vi "DB_Read.vi"(11 "Input Params":T1={"Address IP"="192.168.1.12", "Rack"=0, "Slot "=2, "DB Number"=1, "Start"=0, "Amount"=0}) -> (1 "?":string, 2 "Data":u8[](array[numeric]), 3 "Status":string="No Error")   [LabVIEW 2023]
uses:
  snap7-full-1.4.0/LabVIEW/lib/Snap7.lvlib
panel:
  out "Size Get":i32
  out "Running":bool
  in  "?":bool
  # "DB Get"
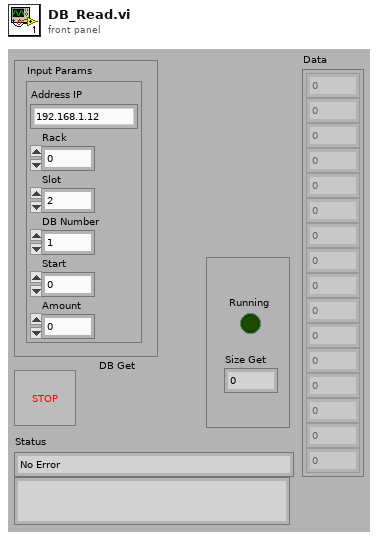
[diagram p1: front panel]
types:
  T1 = cluster{"Address IP":string, "Rack":i32, "Slot ":i32, "DB Number":i32, "Start":i32, "Amount":i32}
  T2 = enum16{"big-endian, network order", "native, host order", "little-endian"}
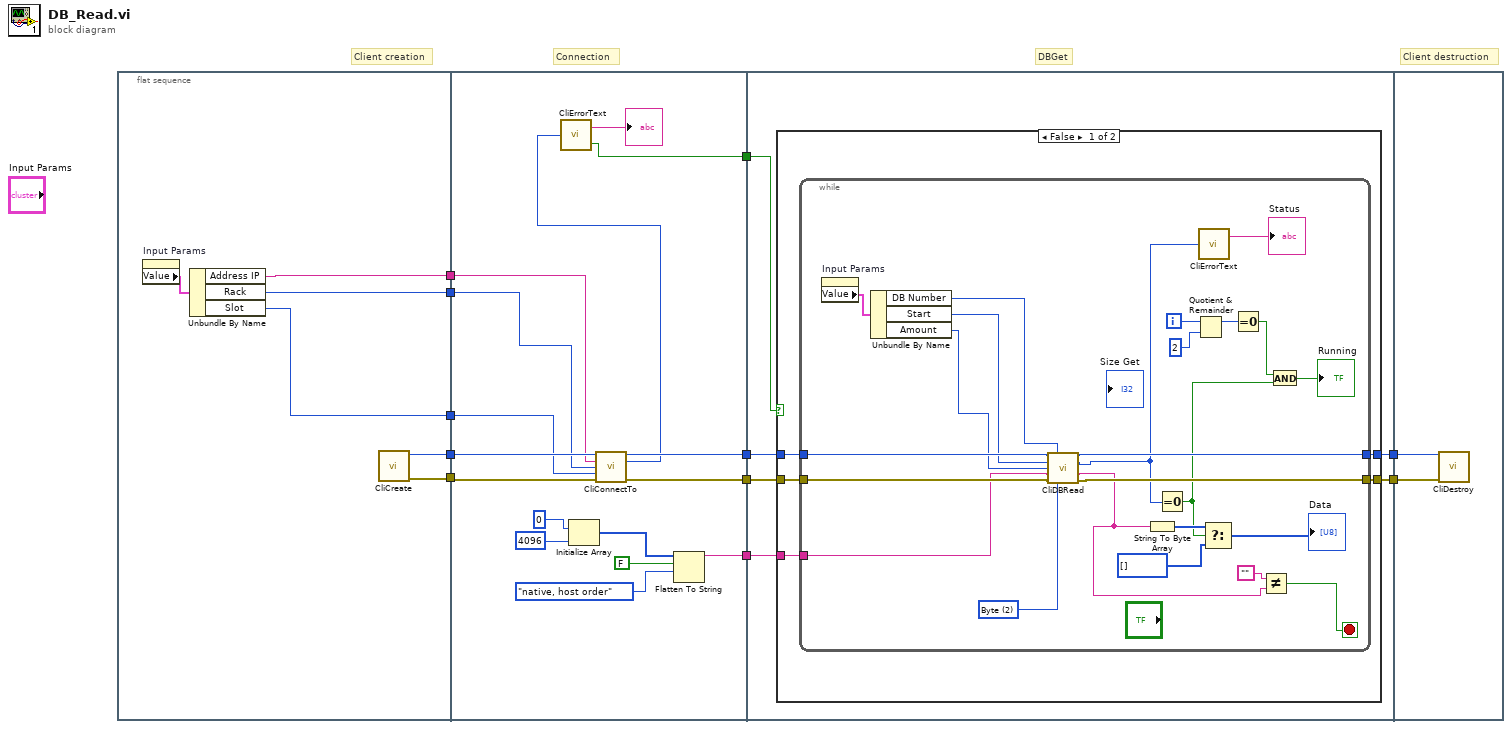
[diagram p0: block diagram]
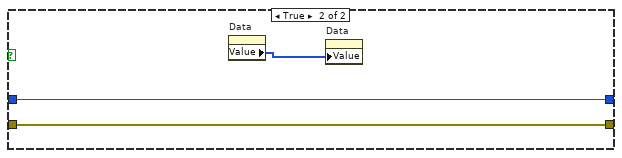
[diagram p2: hidden frame]
diagram:
  # "Client destruction"
  # "DBGet"
  # "Connection"
  # "Client creation"
  n1 = flat-sequence {
    tunnel: [w17] -> w8
    tunnel: [w16] -> w7
    tunnel: [w14] -> w4
    tunnel: [w13] -> w3
    tunnel: [w12] -> w2
    tunnel: [w28] -> w11
    tunnel: [w24] -> w10
    tunnel: [w27] -> w9
    tunnel: w8 -> [w26]
    tunnel: w7 -> [w25]
    tunnel: w4 -> [w21]
    tunnel: w3 -> [w20]
    tunnel: w2 -> [w19]
    tunnel: [w18] -> w1
    tunnel: w11 -> [w39]
    tunnel: w10 -> [w38]
    tunnel: w9 -> [w37]
    tunnel: [w36] -> w6
    tunnel: [w35] -> w5
    tunnel: w1 -> [w34]
    tunnel: w6 -> [w73]
    tunnel: w5 -> [w72]
    frame #0 {
      n2 = property on="Input Params" class="Clust (strict)"() -> ("Value"=w15:T1)  [unwired: 2 in, 2 out]
      n3 = Unbundle By Name(w15) -> ("Address IP"=w14:string, "Rack"=w13:i32, "Slot"=w12:i32)
      n4 = call "CliCreate.vi"() -> ("ref out"=w17:u64, "error out"=w16:errorcluster)  [unwired: 14 in]
    }
    frame #1 {
      n5 = Initialize Array(u8 0, 4096) -> (w31:u8[])
      n6 = call "CliConnectTo.vi"("ref in"=w26, "Address"=w21, "Rack"=w20, "Slot"=w19, "error in (no error)"=w25) -> ("ref out"=w24:u64, "Result"=w23:i32, "error out"=w28:errorcluster)  [unwired: 8 in]
      n7 = call "CliErrorText.vi"("ErrNo"=w23) -> ("Error"=w18:bool, "ErrMessage"=→"?":string)
      n8 = Flatten To String(anything=w31, prepend array or string size? (T)=FALSE, byte order (0:big-endian, network order)=T2."native, host order") -> (data string=w27:string)  [unwired: 1 in, 2 out]
    }
    frame #2 {
      n9 = case shown="False" w34 {
        tunnel: w39 -> [w44 w70]
        tunnel: w38 -> [w43 w71]
        tunnel: w37 -> [w42 _]
        tunnel: [w41 w71] -> w36
        tunnel: [w40 w70] -> w35
        frame False {
          n10 = while {
            tunnel: w44 -> [w60]
            tunnel: w43 -> [w58]
            tunnel: w42 -> [w59]
            tunnel: [w57] -> w41
            tunnel: [w56] -> w40
            i -> [w66]
            stop <- w48 stop-if-true
            w54 = 2 items=["Bit"=1, "Byte"=2, "Word"=4, "DWord"=6, "Real"=8, "Counter"=28, "Timer"=29] ("Word Length")
            n11 = property on="Input Params" class="Clust (strict)"() -> ("Value"=w53:T1)  [unwired: 2 in, 2 out]
            n12 = Unbundle By Name(w53) -> ("DB Number"=w52:i32, "Start"=w51:i32, "Amount"=w50:i32)
            n13 = call "CliDBRead.vi"("ref in"=w58, "DB Number"=w52, "Start"=w51, "Amount"=w50, "data in"=w59, "error in (no error)"=w60, "Word Length"=w54) -> ("ref out"=w57:u64, "Result"=w55:i32, "data out"=w46:string, "error out"=w56:errorcluster)  [unwired: 5 in]
            n14 = String To Byte Array(string=w46) -> (unsigned byte array=w68:u8[])
            n15 = Equal To 0?(x=w55) -> (x = 0?=w49:bool)
            n16 = Quotient & Remainder(x=w66, y=2) -> (x-y*floor(x/y)=w64:i32)  [unwired: 1 out]
            n17 = call "CliErrorText.vi"("ErrNo"=w55) -> ("ErrMessage"=→"Status":string)  [unwired: 1 out]
            n18 = Select(t=w68, s=w49, f=u8[] []) -> (s? t:f=→"Data":u8[])
            n19 = Equal To 0?(x=w64) -> (x = 0?=w63:bool)
            n20 = Not Equal?(x="", y=w46) -> (x != y?=w48:bool)
            n21 = And(x=w63, y=w49) -> (x .and. y?=→"Running":bool)
          }
        }
        frame True {
          n22 = property on="Data" class="Arr (strict)"() -> ("Value"=w69:u8[])  [unwired: 2 in, 2 out]
          n23 = property on="Data" class="Arr (strict)"("Value"=w69) -> ()  [unwired: 2 in, 2 out]
        }
      }
    }
    frame #3 {
      n24 = call "CliDestroy.vi"("ref in"=w73, "error in (no error)"=w72) -> ()  [unwired: 13 in, 1 out]
    }
  }
